vi "Ticks to Inches.vi"(8 "Ticks":dbl, 9 "Wheel revs / gear revs":dbl, 10 "Ticks / gear revs":dbl, 11 "Diameter":dbl) -> (3 "Inches":dbl)   [LabVIEW 2014]
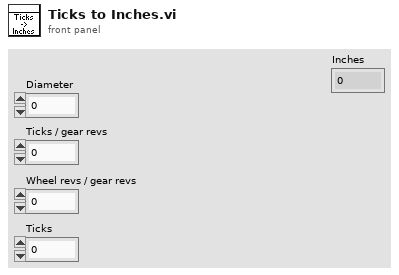
[diagram p1: front panel]
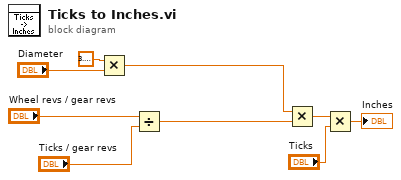
[diagram p0: block diagram]
diagram:
  n1 = Multiply(x=3.141592653589793, y="Diameter") -> (x*y=w5:dbl)
  n2 = Divide(x="Wheel revs / gear revs", y="Ticks / gear revs") -> (x/y=w4:dbl)
  n3 = Multiply(x=w5, y=w4) -> (x*y=w2:dbl)
  n4 = Multiply(x=w2, y="Ticks") -> (x*y=→"Inches":dbl)
